vi "RFmx_An_OBW_Disp.vi"(6 "OBW_Values":dbl[](array[numeric]) format="%#_6p", 9 "CarrierFrequency":dbl format="%#_6p", 10 "SignalBandwidth":dbl format="%#_6p", 11 "Input_Waveform":cluster{"x0":dbl, "dx":dbl, "y":sgl[]}) -> (3 "Waveform Graph 2":cluster{"x0":dbl, "dx":dbl, "y":sgl[]}[](graph))   [LabVIEW 2014]
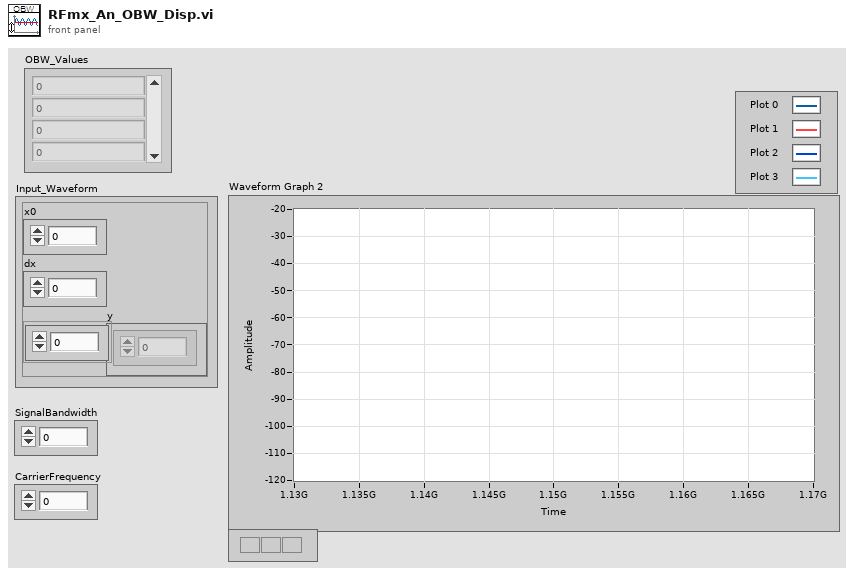
[diagram p1: front panel]
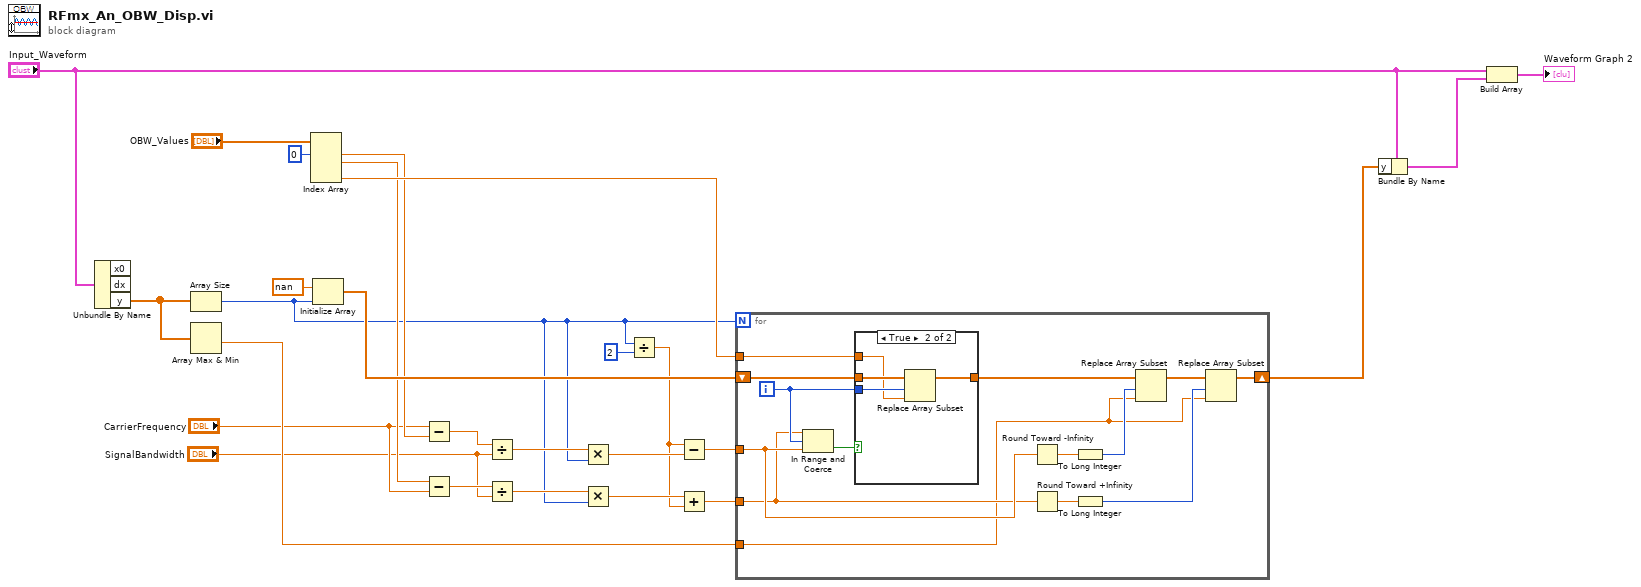
[diagram p0: block diagram]
diagram:
  n1 = Unbundle By Name("Input_Waveform") -> ("y"=w25:sgl[])  [unwired: 2 out]
  n2 = Array Size(array=w25) -> (size(s)=w3:i32)
  n3 = Array Max & Min(array=w25) -> (min value=w19:sgl)  [unwired: 3 out]
  n4 = Index Array(array="OBW_Values", index #1=0 ("index")) -> (element #1=w15:dbl, element #2=w14:dbl, element #4=w16:dbl)  [unwired: 3 in, 1 out]
  n5 = Initialize Array(nan ("element"), w3) -> (w22:dbl[])
  n6 = Subtract(x="CarrierFrequency", y=w15) -> (x-y=w12:dbl)
  n7 = Subtract(x=w14, y="CarrierFrequency") -> (x-y=w11:dbl)
  n8 = Divide(x=w12, y="SignalBandwidth") -> (x/y=w9:dbl)
  n9 = Divide(x=w11, y="SignalBandwidth") -> (x/y=w8:dbl)
  n10 = Multiply(x=w9, y=w3) -> (x*y=w4:dbl)
  n11 = Multiply(x=w8, y=w3) -> (x*y=w7:dbl)
  n12 = Divide(x=w3, y=2) -> (x/y=w1:dbl)
  n13 = Subtract(x=w1, y=w4) -> (x-y=w6:dbl)
  n14 = Add(x=w7, y=w1) -> (x+y=w5:dbl)
  n15 = for {
    N: w3 -> [_]
    shift-right: [w28] -> w18
    shift-left: w22 -> [w40]
    tunnel: w5 -> [w30]
    tunnel: w6 -> [w31]
    tunnel: w19 -> [w29]
    tunnel: w16 -> [w27]
    i -> [w38]
    n16 = In Range and Coerce(upper limit=w30, x=w38, lower limit=w31) -> (In Range?=w39:bool)  [unwired: 1 out]
    n17 = case shown="True" w39 {
      tunnel: w40 -> [w41 w45]
      tunnel: w38 -> [_ w44]
      tunnel: [w41 w43] -> w32
      tunnel: w27 -> [_ w42]
      frame False {
      }
      frame True {
        n18 = Replace Array Subset(array=w45, new element=w42, index=w44) -> (w43:dbl[])
      }
    }
    n19 = Round Toward -Infinity(1:w31) -> (0:w37:dbl)
    n20 = Round Toward +Infinity(x=w30) -> (ceil(x): smallest int >= x=w36:dbl)
    n21 = To Long Integer(number=w37) -> (32bit integer=w35:i32)
    n22 = To Long Integer(number=w36) -> (32bit integer=w33:i32)
    n23 = Replace Array Subset(array=w32, new element=w29, index=w35) -> (w34:dbl[])
    n24 = Replace Array Subset(array=w34, new element=w29, index=w33) -> (w28:dbl[])
  }
  n25 = Bundle By Name(cluster="Input_Waveform", "y"=w18) -> (w17:cluster{"x0":dbl, "dx":dbl, "y":sgl[]})
  n26 = Build Array("Input_Waveform", w17) -> (→"Waveform Graph 2":cluster{"x0":dbl, "dx":dbl, "y":sgl[]}[])
